vi "gu_search_split_string.vi"(7 "Reverse Search (F)":bool, 8 "error in":errorcluster, 9 "Offset (0)":i32, 10 "Encoded String/Codepoint":T1, 11 "Encoded String":T1) -> (0 "error out":errorcluster, 2 "Encoded String B":T1, 3 "Encoded String A":T1)   [LabVIEW 2020, in "G-Unicode.lvlib"]
uses:
  G-Unicode.lvlib
  Types/Encoded UTF-8 String.ctl
  Memory/Copy String.vi/4d47babd-4a2d-4eb7-b91b-7e707d692665.vi
  gu_free.vi
  lib/g_unicode_32.dll
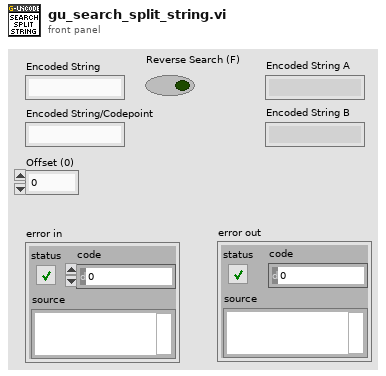
[diagram p1: front panel]
types:
  T1 = typedef "G-Unicode.lvlib/Encoded UTF-8 String.ctl" = string
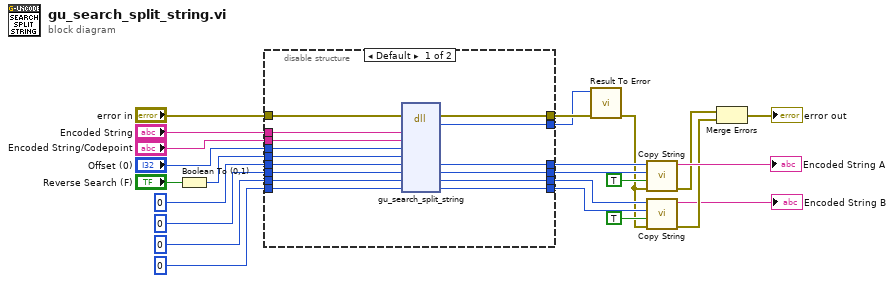
[diagram p0: block diagram]
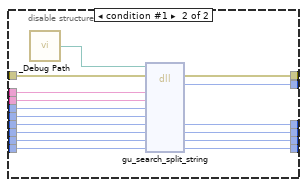
[diagram p2: hidden frame]
diagram:
  n1 = Boolean To (0,1)(Boolean="Reverse Search (F)") -> (0, 1=w9:i16)
  n2 = disable-structure shown="Default" {
    disable-tunnel: "Encoded String" -> [w38 w54]
    disable-tunnel: "error in" -> [w39 w55]
    disable-tunnel: [w37 w53] -> w3
    disable-tunnel: [w36 w52] -> w21
    disable-tunnel: [w35 w51] -> w20
    disable-tunnel: [w34 w50] -> w17
    disable-tunnel: [w33 w49] -> w16
    disable-tunnel: "Encoded String/Codepoint" -> [w32 w48]
    disable-tunnel: w9 -> [w31 w47]
    disable-tunnel: i64 0 ("string_a_pointer") -> [w30 w46]
    disable-tunnel: 0 ("string_a_size") -> [w29 w45]
    disable-tunnel: i64 0 ("string_b_pointer") -> [w28 w44]
    disable-tunnel: 0 ("string_b_size") -> [w27 w43]
    disable-tunnel: "Offset (0)" -> [w26 w41]
    disable-tunnel: [w25 w40] -> w1
    frame condition #0 (active) {
      n3 = dll-call lib="C:/github/dataflowg/g-unicode/src/LabVIEW/G-Unicode/lib/g_unicode_*.*" fn="gu_search_split_string"(error in=w39, "string"=w38, "search_string"=w32, "offset"=w26, "direction"=w31, "string_a_pointer"=w30, "string_a_size"=w29, "string_b_pointer"=w28, "string_b_size"=w27) -> (error out=w37:errorcluster, "result"=w25:i32, "string_a_pointer"=w36:i64, "string_a_size"=w35:i32, "string_b_pointer"=w34:i64, "string_b_size"=w33:i32)  [unwired: 6 in, 1 out]
    }
    frame condition #1 {
      n4 = call "_Debug Path.vi"() -> ("Debug Path"=w42:path)
      n5 = dll-call lib="?" fn="gu_search_split_string"(path in=w42, error in=w55, "string"=w54, "search_string"=w48, "offset"=w41, "direction"=w47, "string_a_pointer"=w46, "string_a_size"=w45, "string_b_pointer"=w44, "string_b_size"=w43) -> (error out=w53:errorcluster, "result"=w40:i32, "string_a_pointer"=w52:i64, "string_a_size"=w51:i32, "string_b_pointer"=w50:i64, "string_b_size"=w49:i32)  [unwired: 5 in, 1 out]
    }
  }
  n6 = call "Result To Error.vi"("error in (no error)"=w3, "Result Code"=w1) -> ("error out"=w2:errorcluster)  [unwired: 9 in]
  n7 = call "Copy String.vi"("error in"=w2, "free (F)"=TRUE, "size"=w20, "pointer"=w21) -> ("error out"=w15:errorcluster, "string"=→"Encoded String A":string)  [unwired: 6 in]
  n8 = call "Copy String.vi"("error in"=w2, "free (F)"=TRUE, "size"=w16, "pointer"=w17) -> ("error out"=w14:errorcluster, "string"=→"Encoded String B":string)  [unwired: 6 in]
  n9 = Merge Errors(w15, w14) -> (→"error out":errorcluster)
